vi "rvc Plot 2D Point.vi"(10 "Y":dbl, 11 "X":dbl) -> (2 "Column vector":dbl[][](array[numeric]), 3 "XY Graph":cluster{dbl[], dbl[]}(graph))   [LabVIEW 2017]
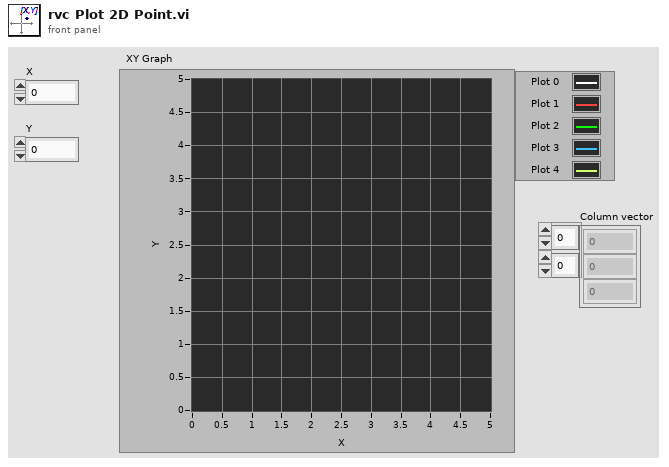
[diagram p1: front panel]
types:
  T1 = typedef "NI_Matrix.lvlib/RealMatrix.ctl" = dbl[][]
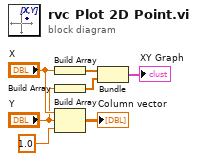
[diagram p0: block diagram]
diagram:
  n1 = Build Array("X") -> (w5:dbl[])
  n2 = Build Array("Y") -> (w6:dbl[])
  n3 = Build Array("X", "Y", 1.0 ("Y")) -> (→"Column vector":T1)
  n4 = Bundle(w5, w6) -> (→"XY Graph":cluster{dbl[], dbl[]})  [unwired: 1 in]
